vi "Initialize Memory Injection Waveform Current.vi"() -> (0 "Init Data Out":fxp<+/-,24,5>[](array[numeric]))   [LabVIEW 2015]
panel:
  out "Waveform Graph":dbl[](graph)
  # "For Initialization VI requirements and help, please read directions located on Block Diagram."
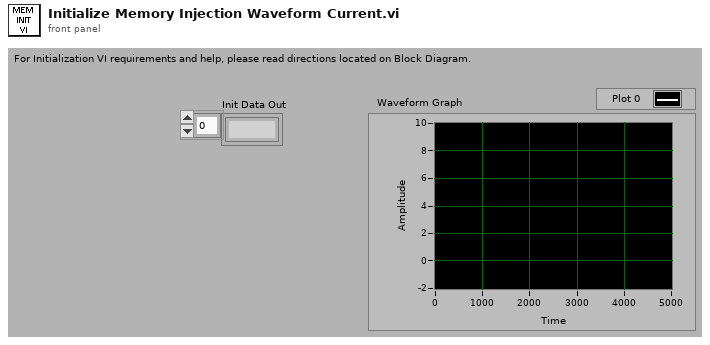
[diagram p1: front panel]
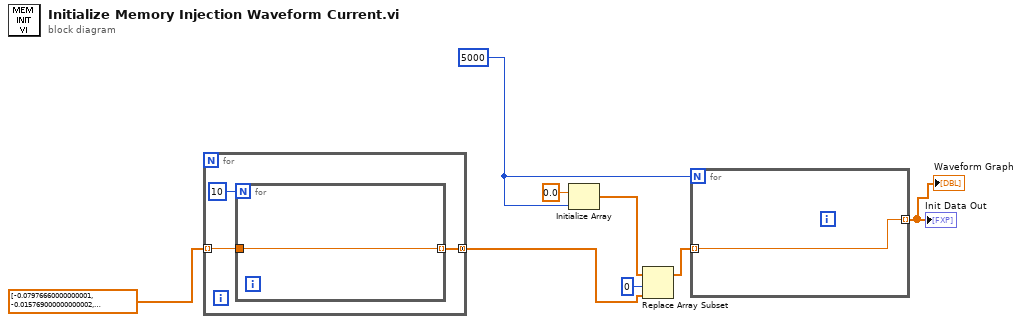
[diagram p0: block diagram]
diagram:
  w8 = 5000 ("Number of Elements")
  n1 = for {
    tunnel: [w11] -> w3 mode=concatenating
    tunnel: dbl[] [-0.07976660000000001, -0.015769000000000002, -0.015769000000000002, -0.143764, -0.07976660000000001, -0.07976660000000001, -0.207762, -0.07976660000000001, -0.07976660000000001, -0.07976660000000001, -0.07976660000000001, -0.07976660000000001, -0.015769000000000002, 0.1762236, 0.1762236, 2.4161400000000004, 4.40006, 6.57598, 8.4319, 6.256, 5.29602, 6.0, 6.51198, 5.4240200000000005, 6.0, 6.319980000000001, 5.4240200000000005, 6.0, 6.57598, 5.616020000000001, 5.29602, 6.256, 6.57598, 5.616020000000001, 5.29602, 6.128, 6.51198, 5.68002, 5.10404, 4.848040000000001, 3.8240800000000004, 4.0160800000000005, 4.33606, 3.8880800000000004, 4.20806, 4.0160800000000005, 4.080080000000001, 4.52806, 4.0160800000000005, 4.65606, 4.080080000000001, 4.52806, 3.7600800000000003, 4.27206, 4.40006, 4.0160800000000005, 4.65606, 3.9520800000000005, 4.46406, 3.8240800000000004, 4.20806, 4.33606, 4.144080000000001, 4.78404, 3.9520800000000005, 4.33606, 4.080080000000001, 4.080080000000001, 4.65606, 3.9520800000000005, 4.59206, 3.7600800000000003, 4.27206, 4.46406, 4.144080000000001, 4.72004, 3.8240800000000004, 4.65606, 3.9520800000000005, 4.33606, 3.8880800000000004, 4.144080000000001, 4.27206, 4.20806, 4.72004, 3.8240800000000004, 4.52806, 4.0160800000000005, 4.20806, 4.27206, 4.080080000000001, 4.65606, 4.0160800000000005, 4.52806, 3.8880800000000004, 4.20806, 4.46406, 4.080080000000001, 4.59206, 4.080080000000001, 4.59206, 3.6960800000000003, 4.27206, 4.080080000000001, 4.20806, 4.59206, 3.8880800000000004, 4.65606, 3.8880800000000004, 4.27206, 4.33606, 4.080080000000001, 4.59206, 3.9520800000000005, 4.72004, 3.8240800000000004, 4.33606, 4.144080000000001, 4.144080000000001, 4.52806, 3.9520800000000005, 4.59206, 1.968154, -0.335756, -0.015769000000000002, -0.143764, -0.143764, -0.207762, -0.143764, -0.143764] ("Current Input Graph 2") -> [w10] mode=indexing
    n2 = for {
      N: 10 -> [_]
      tunnel: [w12] -> w11 mode=indexing
      tunnel: w10 -> [w12]
    }
  }
  n3 = Initialize Array(0.0 ("element"), w8) -> (w6:dbl[])
  n4 = Replace Array Subset(array=w6, new element=w3, index=0) -> (w4:dbl[])
  n5 = for {
    N: w8 -> [_]
    tunnel: [w13] -> w2 mode=indexing
    tunnel: w4 -> [w13] mode=indexing
  }
  "Init Data Out" <- w2
  "Waveform Graph" <- w2
